vi "VI Analyser.vi"() -> ()   [LabVIEW 2020]
uses:
  <vilib>/addons/analyzer/NI_VIAnalyzerTKVIs.lvlib
panel:
  out "Analysis Progress":dbl(slide) scale=0.0..100.0
  out "VI in Analysis":string
  out "Tests Run":string[](array[string])
  out "VIs Tested":path[](array[path])
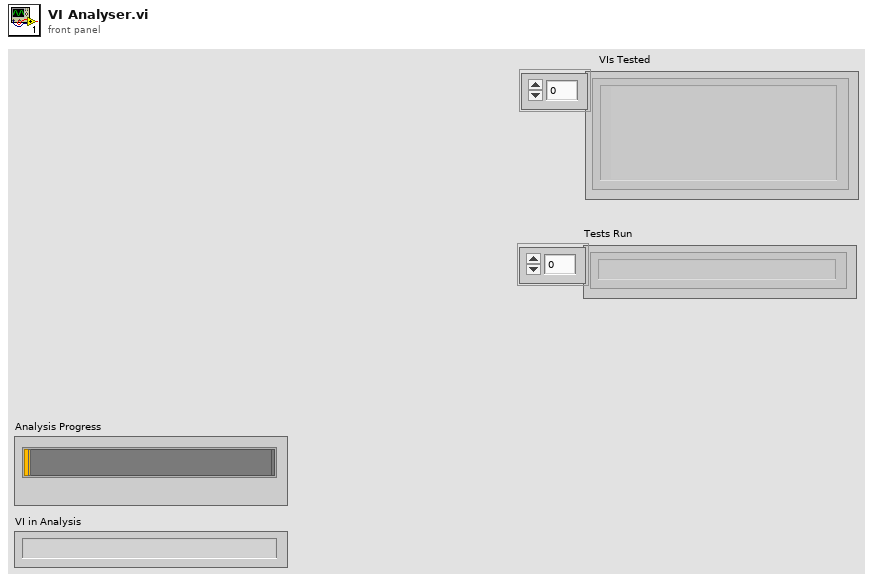
[diagram p1: front panel]
types:
  T1 = typedef "VIAnAPI Ref.ctl" = refnum<k1>
  T2 = typedef "VIAnCtl Results.ctl" = cluster{"Test Name":string, "Results Data":T3[], "Status":T4, "Exceed Max Fails?":bool}
  T3 = typedef "VIAnCtl ResultsData (index).ctl" = cluster{"Result Message":string, "Ref Index":i32}
  T4 = typedef "VIAnCtl ResultStatus.ctl" = enum16{"Pass", "Fail", "Skipped", "VI not loadable", "Test not loadable", "Test not runnable", "Test error out"}
  T5 = typedef "VIAnRes Parsed Results Data (by VI).ctl" = cluster{"VI Path":path, "Pass":cluster{"row":i32, "column":i32}[], "Fail":cluster{"row":i32, "column":i32}[], "Skipped":cluster{"row":i32, "column":i32}[], "VI not loadable":cluster{"row":i32, "column":i32}[], "Test not loadable":cluster{"row":i32, "column":i32}[], "Test not runnable":cluster{"row":i32, "column":i32}[], "Test error out":cluster{"row":i32, "column":i32}[]}
  T6 = typedef "VIAnRes Parsed Results Data (by Test).ctl" = cluster{"Test Name":string, "Pass":cluster{"VI Path":path, "index":cluster{"row":i32, "column":i32}}[], "Fail":cluster{"VI Path":path, "index":cluster{"row":i32, "column":i32}}[], "Skipped":cluster{"VI Path":path, "index":cluster{"row":i32, "column":i32}}[]}
  T7 = typedef "VIAnCtl Test Config Data.ctl" = cluster{"Test Name":string, "Config Ref":refnum<vi>, "Ref Valid?":bool, "Test Ranking":T8, "Max Failures":u32, "Test Path":path, "Control Values":T9[], "Selected?":bool}
  T8 = typedef "VIAnCtl TestRanking.ctl" = u16
  T9 = typedef "VIAnCtl Config Control Value.ctl" = cluster{"Control Name":string, "Control Value":variant}
  T10 = cluster{"Raw Results":T2[][], "Parsed Results Data (by VI)":T5[], "Parsed Results Data (by Test)":T6[], "Summary Statistics":cluster{"Passed Tests":i32, "Failed Tests":i32, "Skipped Tests":i32, "VIs not loadable":i32, "Tests not loadable":i32, "Tests not runnable":i32, "Test error out":i32, "Start Time":u32, "Total Time (s)":dbl}, "Test Config Data":T7[]}
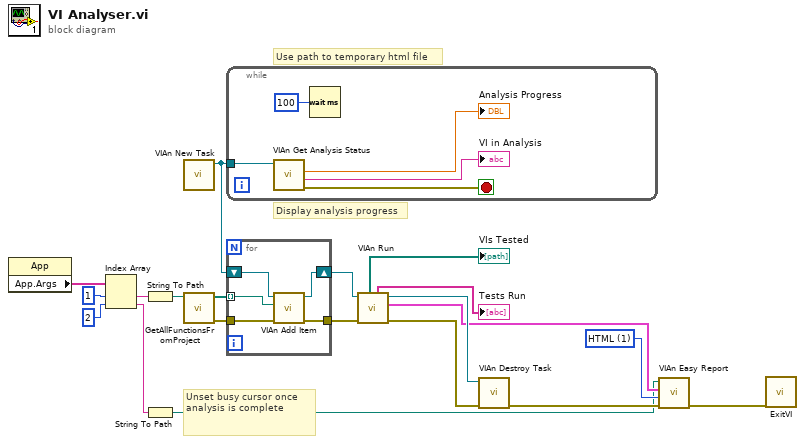
[diagram p0: block diagram]
diagram:
  w17 = u16 1 items=["ASCII", "HTML", "RSL File"] ("Report Save Type (ASCII)")
  # "Display analysis progress"
  # "Unset busy cursor once analysis is complete"
  # "Use path to temporary html file"
  n1 = property class="App"() -> ("App.Args"=w4:string[])  [unwired: 2 in, 2 out]
  n2 = Index Array(array=w4, index #1=1 ("index"), index #2=2 ("index")) -> (element #1=w8:string, element #2=w7:string)
  n3 = String To Path(string=w8) -> (path=w3:path)
  n4 = String To Path(string=w7) -> (path=w2:path)
  n5 = call <vilib>:"VIAn New Task.vi"() -> ("VI Analyzer Task"=w11:T1)  [unwired: 10 in, 1 out]
  n6 = call "GetAllFunctionsFromProject.vi"("Path"=w3) -> ("error out"=w9:errorcluster, "MethodPaths"=w10:path[])  [unwired: 9 in]
  n7 = while {
    tunnel: w11 -> [w25]
    stop <- w21 stop-if-true
    n8 = call <vilib>:"VIAn Get Analysis Status.vi"("VI Analyzer Task in"=w25) -> ("error out"=w21:errorcluster, "VI in Analysis"=→"VI in Analysis":string, "Percent Complete"=→"Analysis Progress":dbl)  [unwired: 1 in, 7 out]
    n9 = Wait (ms)(milliseconds to wait=u32 100) -> ()  [unwired: 1 out]
  }
  n10 = for {
    tunnel: w10 -> [w29] mode=indexing
    tunnel: w9 -> [w27]
    shift-right: [w28] -> w14
    shift-left: w11 -> [w30]
    tunnel: [w26] -> w12
    n11 = call <vilib>:"VIAn Add Item.vi"("error in (no error)"=w27, "Item to Add"=w29, "VI Analyzer Task in"=w30) -> ("error out"=w26:errorcluster, "VI Analyzer Task out"=w28:T1)  [unwired: 7 in]
  }
  n12 = call <vilib>:"VIAn Run.vi"("error in (no error)"=w12, "VI Analyzer Task in"=w14) -> ("error out"=w13:errorcluster, "Analysis Results"=w18:T10, "VI Analyzer Task out"=w20:T1, "Tests Run"=→"Tests Run":string[], "VIs Tested"=→"VIs Tested":path[])  [unwired: 5 out]
  n13 = call <vilib>:"VIAn Destroy Task.vi"("error in (no error)"=w13, "VI Analyzer Task in"=w20) -> ("error out"=w19:errorcluster)  [unwired: 9 out]
  n14 = call <vilib>:"VIAn Easy Report.vi"("error in (no error)"=w19, "Report Save Type (ASCII)"=w17, "Analysis Results"=w18, "Report Save Path"=w2) -> ("error out"=w1:errorcluster)  [unwired: 3 in, 4 out]
  n15 = call "ExitVI.vi"("error in (no error)"=w1) -> ()  [unwired: 10 in, 1 out]
